vi "ReturnsCorrectLoyaltyDiscountForLongtimeCustomers.vi"(8 "Error In":errorcluster, 9 "ExpectedDiscount":ext, 10 "YearsAsCustomer":i32, 11 "reference in":refnum<class "DiscountCalculator_CalculateDiscountPercentage.lvclass">) -> (0 "Error Out":errorcluster, 3 "reference out":refnum<class "DiscountCalculator_CalculateDiscountPercentage.lvclass">)   [LabVIEW 2020, in "DiscountCalculator_CalculateDiscountPercentage.lvclass"]
uses:
  DiscountCalculator_CalculateDiscountPercentage.lvclass
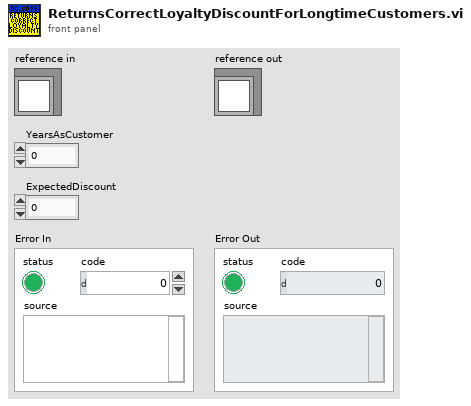
[diagram p1: front panel]
types:
  T1 = typedef "DiscountCalculator_CalculateDiscountPercentage.lvclass/ObjectAttributes.ctl" = cluster{"_calculator":refnum<class "DiscountCalculator.lvclass">, "DEFAULT_AGE":i32}
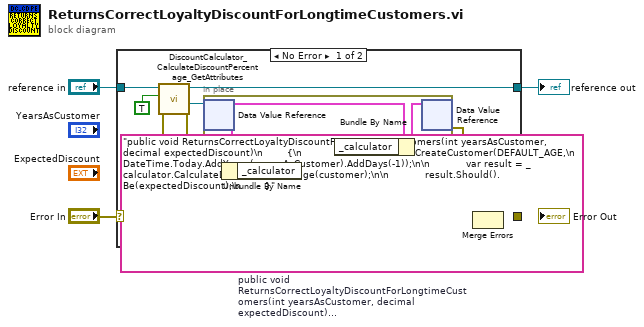
[diagram p0: block diagram]
diagram:
  (unwired) "public void ReturnsCorrectLoyaltyDiscountForLongtimeCustomers(int yearsAsCustomer, decimal expectedDiscount)\n        {\n            var customer = CreateCustomer(DEFAULT_AGE,\n                DateTime.Today.AddYears(-yearsAsCustomer).AddDays(-1));\n\n            var result = _calculator.CalculateDiscountPercentage(customer);\n\n            result.Should().Be(expectedDiscount);\n        }"  # public void ReturnsCorrectLoyaltyDiscountForLongtimeCustomers(int yearsAsCustomer, decimal expectedDiscount)         {             var customer = CreateCustomer(DEFAULT_AGE,                 DateTime.Today.AddYears(-yearsAsCustomer).AddDays(-1));              var result = _calculator.CalculateDiscountPercentage(customer);              result.Should().Be(expectedDiscount);         }
  n1 = case shown="No Error" "Error In" {
    selector: "Error In" -> [w11 w16]
    tunnel: [w8 w16] -> w3
    tunnel: [w9 w15] -> w1
    tunnel: "reference in" -> [w12 w15]
    frame No Error {
      n2 = call "DiscountCalculator_CalculateDiscountPercentage_GetAttributes.vi"("error in (no error)"=w11, "OnlyGetDvrReference(False)"=TRUE, "reference in"=w12) -> ("error out"=w6:errorcluster, "DataRef"=w7:refnum<data-value>, "reference out"=w9:refnum<class "DiscountCalculator_CalculateDiscountPercentage.lvclass">)  [unwired: 5 in, 1 out]
      n3 = in-place {
        n4 = in-place-dvr #1(w7) -> (w13:T1)  [unwired: 1 out]
        n5 = Unbundle By Name(w13) -> ()  [unwired: 1 out]
        n6 = Bundle By Name(cluster=w13) -> (w14:T1)  [unwired: 1 in]
        n7 = in-place-dvr #1(w14) -> (w10:errorcluster)  [unwired: 1 out]
      }
      n8 = Merge Errors(w6, w10) -> (w8:errorcluster)
    }
    frame Error {
    }
  }
  "Error Out" <- w3
  "reference out" <- w1
